vi "Stiffness Test.vi"(6 "Limits":dbl[](array[numeric]), 9 "Prev Stiffness Value":dbl, 10 "Stiffness Value In":dbl) -> (2 "Stiffness Value Out":dbl)   [LabVIEW 2013]
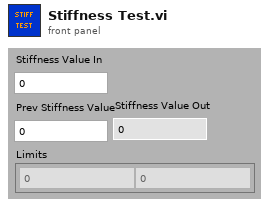
[diagram p1: front panel]
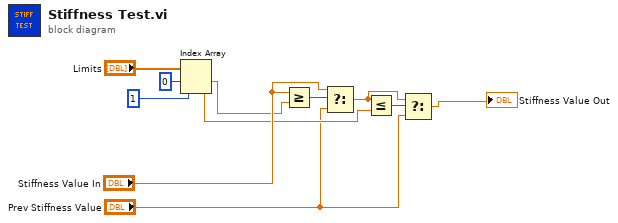
[diagram p0: block diagram]
diagram:
  n1 = Index Array(array="Limits", index #1=0 ("index"), index #2=1 ("index")) -> (element #1=w6:dbl, element #2=w3:dbl)
  n2 = Greater Or Equal?(x="Stiffness Value In", y=w6) -> (x >= y?=w8:bool)
  n3 = Select(t="Stiffness Value In", s=w8, f="Prev Stiffness Value") -> (s? t:f=w4:dbl)
  n4 = Less Or Equal?(x=w4, y=w3) -> (x <= y?=w5:bool)
  n5 = Select(t=w4, s=w5, f="Prev Stiffness Value") -> (s? t:f=→"Stiffness Value Out":dbl)
